vi "RealTime.vi"() -> ()   [LabVIEW 2019]
uses:
  <vilib>/Bytelabs/ByteTCP/TCP_Class/TCP.lvclass
  TypeDef/TCPMessage.ctl
  <vilib>/Bytelabs/ByteSimpleQ/ByteSimpleQ/ByteSimpleQ.lvlib
  TypeDef/ChannelInfo.ctl
  bytetcp/TCPLib/TCP_Class/TCP.lvclass
  <vilib>/Bytelabs/ByteChannelsSetting/ChannelSettingsLib/ChannelsRepos/ChannelsRepoXML/ChannelsRepoXML.lvclass
  source/ByteQXAPIBase/LimsTestStep/acquisitions.ctl
  source/ByteQXAPIBase/ByteQXAPIBase.lvclass
  <vilib>/Utility/xml.llb/Write to XML File(string).vi
  source/ByteQXAPIBase/TypeDef/Step.ctl
  source/ByteQXAPIBase/UpdateChannelsList/fields.ctl
  source/ByteQXAPIBase/TypeDef/Asset.ctl
panel:
  out "error out":errorcluster
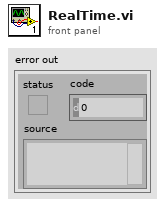
[diagram p1: front panel]
types:
  T1 = typedef "ChannelInfo.ctl" = cluster{"Tag":string, "HW Resource":string, "Raw":dbl}
  T2 = typedef "ByteQXWebAPI.lvlib/ByteQXAPIBase.lvclass/acquisitions.ctl" = cluster{"tags":cluster{"step_id":i32, "test_slug":string, "asset_slug":string}, "acquisitions":cluster{"timestamp":string, "fields":cluster{"name":string, "value":dbl}[]}[]}
  T3 = cluster{"queue out":refnum<queue>, "Acquisitions":T2, "Info":T1[], "TCP_Class":refnum<class "TCP.lvclass">, "Continous?":bool, "Duration":dbl}
  T4 = cluster{"ByteGSAPIBase in":refnum<class "ByteQXAPIBase.lvclass">, "TCP_Class":refnum<class "TCP.lvclass">, "ChannelsRepoBase out":refnum<class "ChannelsRepoXML.lvclass">, "queue out":refnum<queue>}
  T5 = cluster{"ChannelsRepoBase out":refnum<class "ChannelsRepoXML.lvclass">, "channels":string[], "Duration":dbl, "id":i32, "prova.slug":string, "Continous?":bool}
  T6 = cluster{"timestamp":string, "fields":cluster{"name":string, "value":dbl}[]}
  T7 = typedef "TCPMessage.ctl" = cluster{"Message":string, "Data":variant}
  T8 = cluster{"timestamp":string, "fields":cluster{"name":string, "value":dbl}[]}[]
  T9 = typedef "ByteQXWebAPI.lvlib/ByteQXAPIBase.lvclass/fields.ctl" = cluster{"asset_slug":string, "fields":string[]}
  T10 = typedef "ByteQXWebAPI.lvlib/ByteQXAPIBase.lvclass/Step.ctl" = cluster{"id":i32, "descrizione":string, "prova":cluster{"slug":string}, "assets":T11[], "criterio_accettazione":string, "valore_criterio_accettazione_max":dbl, "valore_criterio_accettazione_min":dbl, "udm_criterio_accettazione":string, "duration_prova":string, "udm_duration_prova":string, "valore_prova":dbl, "ordine":i32, "user":i32, "link_automation":string, "instruction_automation":string, "data_completamento_checklist":timestamp, "outcome":bool, "step_type":string, "channels":string[]}
  T11 = typedef "ByteQXWebAPI.lvlib/ByteQXAPIBase.lvclass/Asset.ctl" = cluster{"descrizione":string, "slug":string, "id":i32}
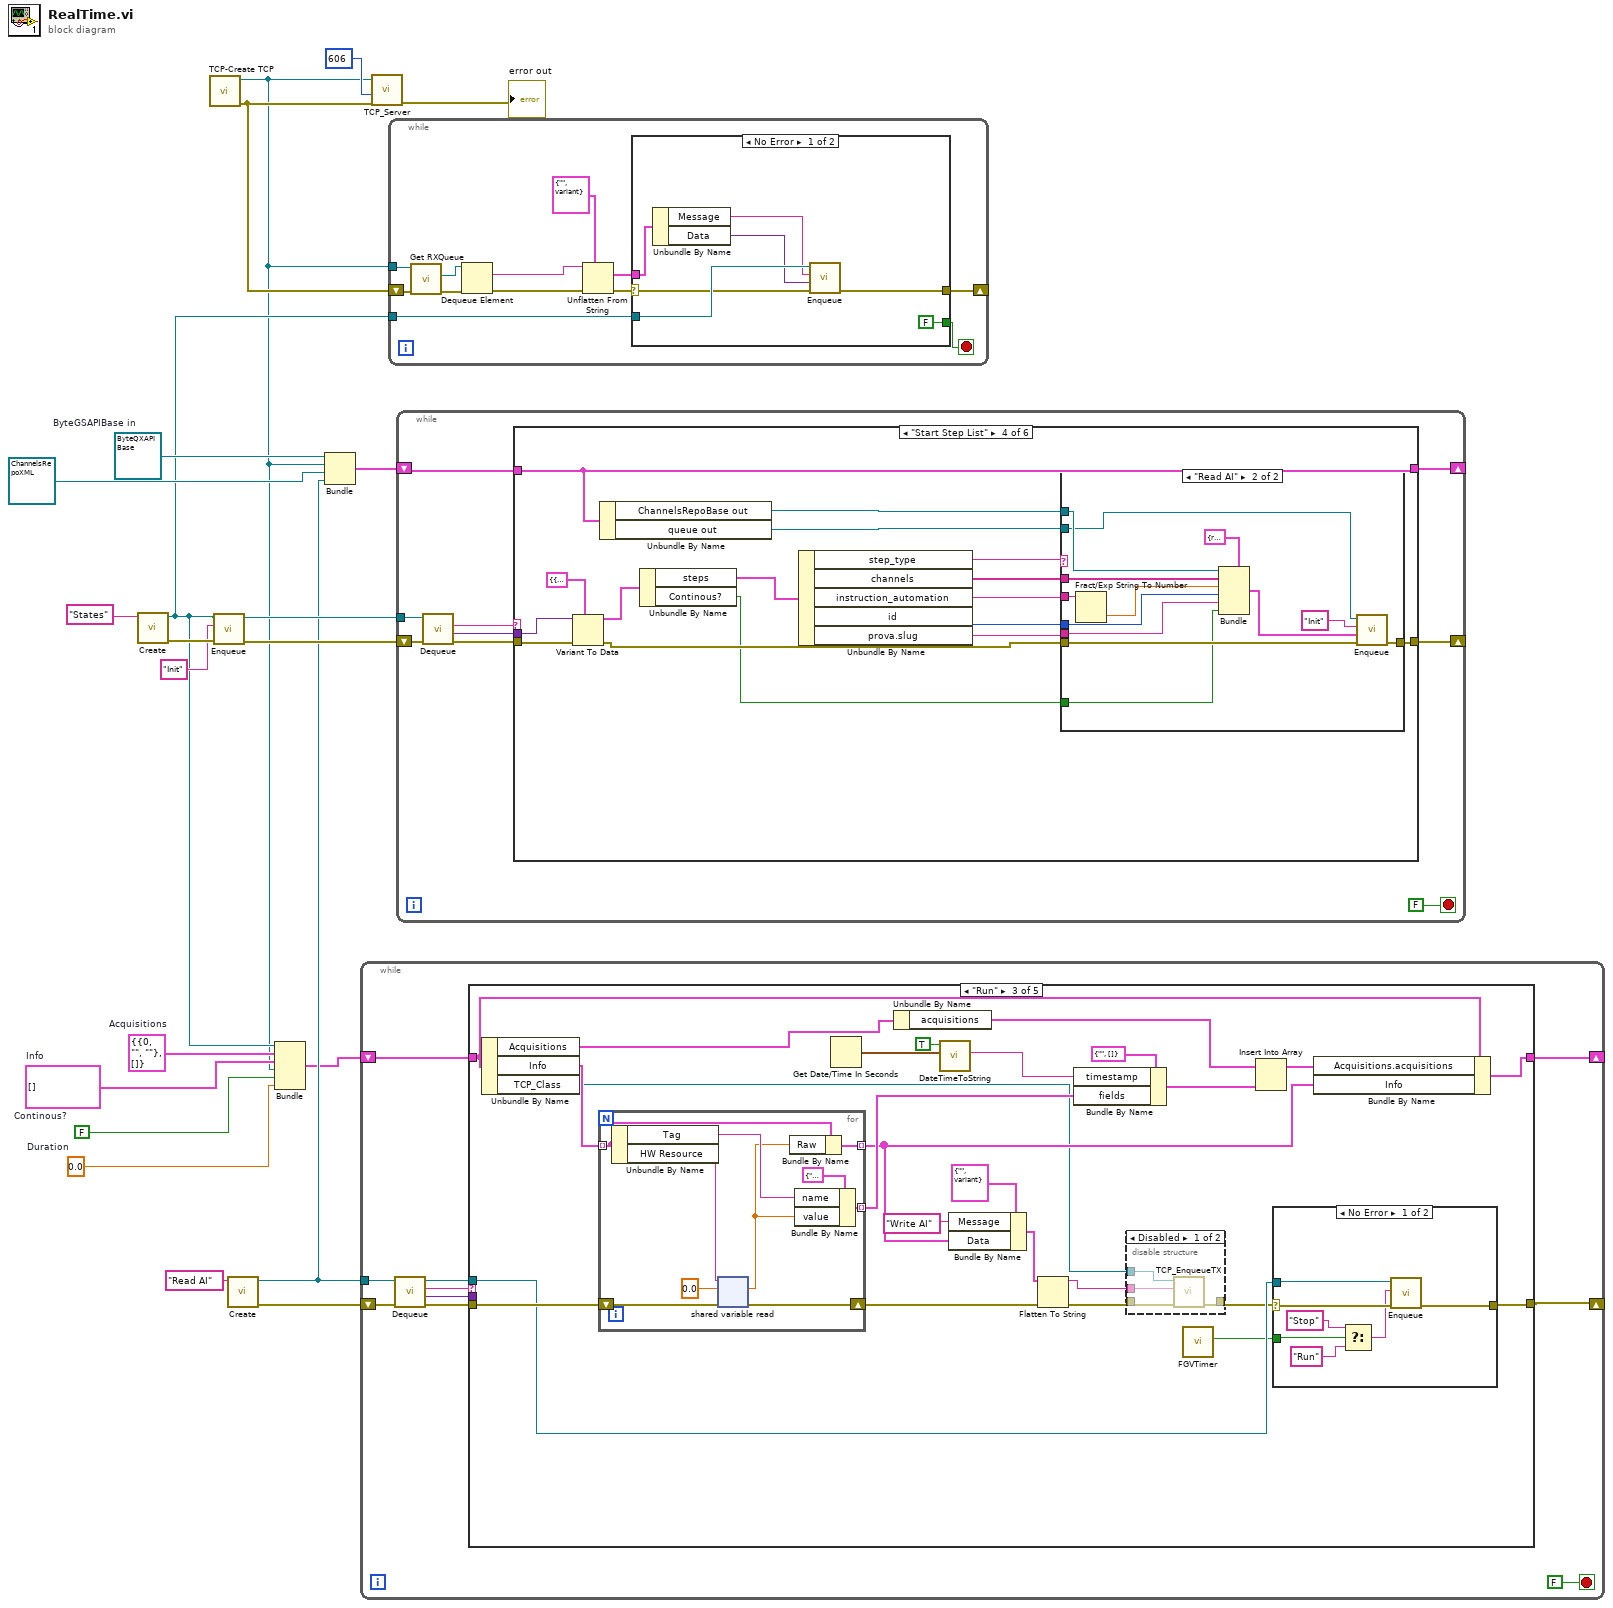
[diagram p0: block diagram]
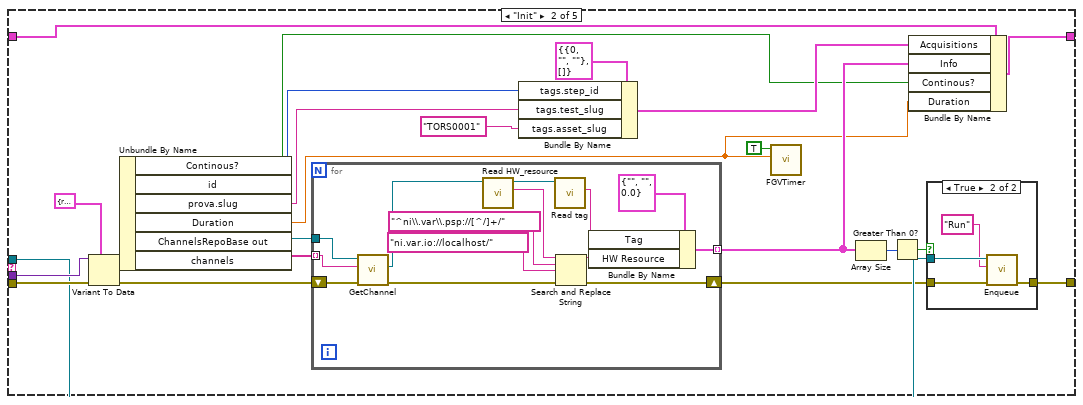
[diagram p3: hidden frame]
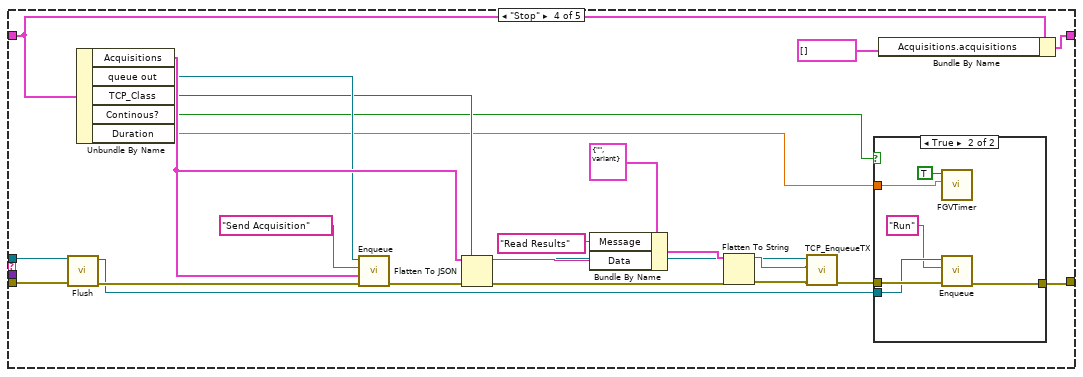
[diagram p7: hidden frame]
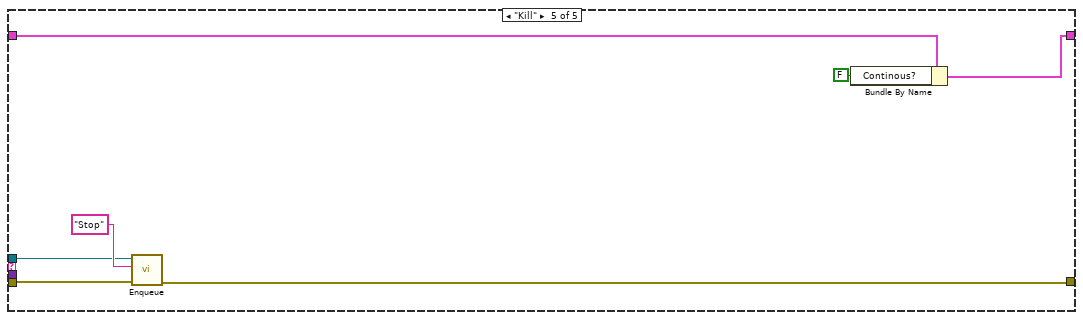
[diagram p9: hidden frame]
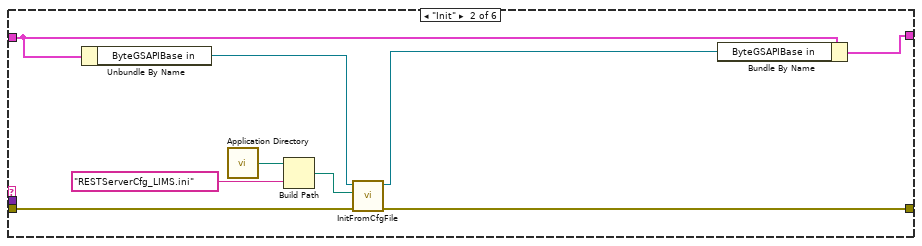
[diagram p11: hidden frame]
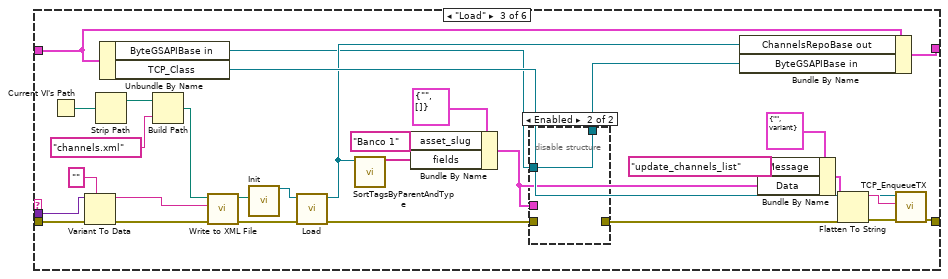
[diagram p12: hidden frame]
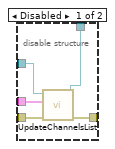
[diagram p13: hidden frame]
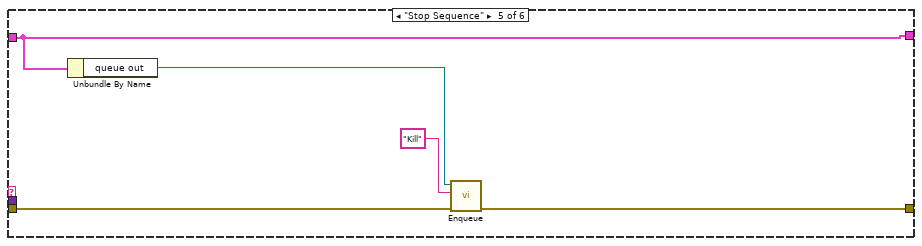
[diagram p15: hidden frame]
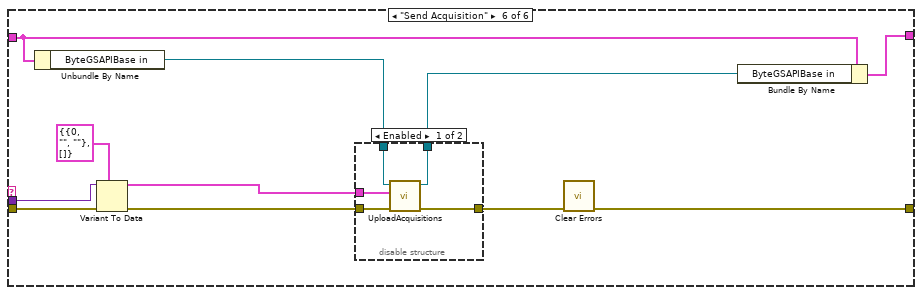
[diagram p16: hidden frame]
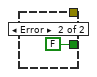
[diagram p18: hidden frame]
diagram:
  w1 = 0.0  # Duration
  w2 = FALSE  # Continous?
  w5 = T1[] []  # Info
  w6 = T2 {"tags"={"step_id"=0, "test_slug"="", "asset_slug"=""}, "acquisitions"=[]}  # Acquisitions
  w11 = refnum<class "ByteQXAPIBase.lvclass"> refnum  # ByteGSAPIBase in
  n1 = call <vilib>:"Create.vi"("name (unnamed)"="States") -> ("error out"=w15:errorcluster, "queue out"=w7:refnum<queue>)  [unwired: 8 in, 1 out]
  n2 = call <vilib>:"TCP-Create TCP.vi"() -> ("error out"=w21:errorcluster, "TCP_Class"=w4:refnum<class "TCP.lvclass">)  [unwired: 9 in, 1 out]
  n3 = call <vilib>:"Enqueue.vi"("error in (no error)"=w15, "message"="Init", "queue in"=w7) -> ("error out"=w14:errorcluster, "queue out"=w13:refnum<queue>)  [unwired: 6 in, 1 out]
  n4 = call <vilib>:"Create.vi"("name (unnamed)"="Read AI") -> ("error out"=w17:errorcluster, "queue out"=w9:refnum<queue>)  [unwired: 8 in, 1 out]
  n5 = Bundle("queue out"=w7, "Acquisitions"=w6, "Info"=w5, "TCP_Class"=w4, "Continous?"=w2, "Duration"=w1) -> (w3:T3)  [unwired: 1 in]
  n6 = Bundle("ByteGSAPIBase in"=w11, "TCP_Class"=w4, "ChannelsRepoBase out"=refnum<class "ChannelsRepoXML.lvclass"> refnum, "queue out"=w9) -> (w8:T4)  [unwired: 1 in]
  n7 = while {
    tunnel: w9 -> [w31]
    shift-right: [w25] -> _
    shift-left: w17 -> [w30]
    shift-right: [w22] -> _
    shift-left: w3 -> [w23]
    stop <- FALSE stop-if-true
    n8 = call <vilib>:"Dequeue.vi"("error in (no error)"=w30, "queue in"=w31) -> ("error out"=w29:errorcluster, "data"=w27:variant, "message"=w28:string, "queue out"=w26:refnum<queue>)  [unwired: 5 in, 1 out]
    n9 = case shown="\"Run\"" w28 {
      tunnel: w29 -> [w33 w56 w100 w145 w158]
      tunnel: w27 -> [_ w55 _ _ _]
      tunnel: w26 -> [_ w51 w99 w144 w157]
      tunnel: [w33 w50 w98 w128 w156] -> w25
      tunnel: w23 -> [w32 w41 w79 w125 w155]
      tunnel: [w32 w39 w77 w124 w153] -> w22
      frame Default {
      }
      frame "Init" {
        n10 = Variant To Data(error in=w56, type=T5 {"ChannelsRepoBase out"=refnum, "channels"=[], "Duration"=0.0, "id"=0, "prova.slug"="", "Continous?"=FALSE} ("output cluster"), Variant=w55) -> (data=w49:T5, error out=w54:errorcluster)
        n11 = Unbundle By Name(w49) -> ("Continous?"=w36:bool, "id"=w43:i32, "prova.slug"=w42:string, "Duration"=w34:dbl, "ChannelsRepoBase out"=w47:refnum<class "ChannelsRepoXML.lvclass">, "channels"=w48:string[])
        n12 = for {
          shift-right: [w70] -> w46
          shift-left: w54 -> [w65]
          tunnel: [w67] -> w38 mode=indexing
          tunnel: w48 -> [w63] mode=indexing
          tunnel: w47 -> [w66]
          n13 = call <vilib>:"GetChannel.vi"("error in (no error)"=w65, "tag"=w63, "ChannelsRepoBase in"=w66) -> ("error out"=w64:errorcluster, "channel"=w62:refnum<class "ChannelBase.lvclass">)  [unwired: 5 in, 2 out]
          n14 = call <vilib>:"Read HW_resource.vi"("ChannelBase in"=w62) -> ("HW_resource"=w75:string, "ChannelBase out"=w72:refnum<class "ChannelBase.lvclass">)  [unwired: 9 in]
          n15 = call <vilib>:"Read tag.vi"("ChannelBase in"=w72) -> ("tag"=w71:string)  [unwired: 9 in, 1 out]
          n16 = Search and Replace String(input string=w75, search string="^ni\\.var\\.psp://[^/]+/", replace string="ni.var.io://localhost/" ("replace string (\"\")"), error in=w64) -> (result string=w69:string, error out=w70:errorcluster)  [unwired: 4 in, 2 out]
          n17 = Bundle By Name(cluster=T1 {"Tag"="", "HW Resource"="", "Raw"=0.0} ("output cluster"), "Tag"=w71, "HW Resource"=w69) -> (w67:T1)
        }
        n18 = Bundle By Name(cluster=T2 {"tags"={"step_id"=0, "test_slug"="", "asset_slug"=""}, "acquisitions"=[]} ("Cluster"), "tags.step_id"=w43, "tags.test_slug"=w42, "tags.asset_slug"="TORS0001") -> (w40:T2)
        n19 = call "FGVTimer.vi"("set timer"=w34, "Reset"=TRUE) -> ()  [unwired: 8 in, 2 out]
        n20 = Array Size(array=w38) -> (size(s)=w53:i32)
        n21 = Greater Than 0?(x=w53) -> (x > 0?=w52:bool)
        n22 = Bundle By Name(cluster=w41, "Acquisitions"=w40, "Info"=w38, "Continous?"=w36, "Duration"=w34) -> (w39:T3)
        n23 = case shown="True" w52 {
          tunnel: w51 -> [_ w61]
          tunnel: [w57 w59] -> w50
          tunnel: w46 -> [w57 w58]
          frame False {
          }
          frame True {
            n24 = call <vilib>:"Enqueue.vi"("error in (no error)"=w58, "message"="Run", "queue in"=w61) -> ("error out"=w59:errorcluster)  [unwired: 6 in, 2 out]
          }
        }
      }
      frame "Run" {
        n25 = Unbundle By Name(w79) -> ("Acquisitions"=w80:T2, "Info"=w81:T1[], "TCP_Class"=w76:refnum<class "TCP.lvclass">)
        n26 = for {
          shift-right: [w118] -> w87
          shift-left: w100 -> [w122]
          tunnel: w81 -> [w119] mode=indexing
          tunnel: [w117] -> w78 mode=indexing
          tunnel: [w114] -> w93 mode=indexing
          n27 = Unbundle By Name(w119) -> ("Tag"=w115:string, "HW Resource"=w120:string)
          n28 = shared-variable-read(w120, w122, 0.0) -> (w118:errorcluster, w113:dbl)  [unwired: 2 out]
          n29 = Bundle By Name(cluster=w119, "Raw"=w113) -> (w117:T1)
          n30 = Bundle By Name(cluster=cluster{"name":string, "value":dbl} {"name"="", "value"=0.0} ("fields"), "name"=w115, "value"=w113) -> (w114:cluster{"name":string, "value":dbl})
        }
        n31 = Get Date/Time In Seconds() -> (seconds since 1Jan1904=w84:timestamp)
        n32 = Unbundle By Name(w80) -> ("acquisitions"=w91:T8)
        n33 = call "DateTimeToString.vi"("current time"=w84, "include Time?"=TRUE) -> ("date string"=w83:string)  [unwired: 8 in, 1 out]
        n34 = Bundle By Name(cluster=T7 {"Message"="", "Data"=variant}, "Message"="Write AI", "Data"=w78) -> (w96:T7)
        n35 = Flatten To String(anything=w96, error in (no error)=w87) -> (data string=w88:string, error out=w89:errorcluster)  [unwired: 2 in, 1 out]
        n36 = Bundle By Name(cluster=T6 {"timestamp"="", "fields"=[]} ("acquisition"), "timestamp"=w83, "fields"=w93) -> (w92:T6)
        n37 = disable-structure shown="Disabled" {
          disable-tunnel: w89 -> [w104 _]
          disable-tunnel: w88 -> [w103 _]
          disable-tunnel: [w102 _] -> w85
          disable-tunnel: w76 -> [w101 _]
          frame Disabled {
            n38 = call-dynamic "TCP_EnqueueTX.vi"("error in (no error)"=w104, "Msg to Transmit"=w103, "TCP in"=w101) -> ("error out"=w102:errorcluster)  [unwired: 7 in, 1 out]
          }
          frame Enabled {
          }
        }
        n39 = call "FGVTimer.vi"() -> ("Elapsed?"=w86:bool)  [unwired: 10 in, 1 out]
        n40 = Insert Into Array(array=w91, new element=w92) -> (w90:T8)  [unwired: 1 in]
        n41 = case shown="No Error" w85 {
          selector: w85 -> [w111 w112]
          tunnel: w99 -> [w109 _]
          tunnel: [w110 w112] -> w98
          tunnel: w86 -> [w108 _]
          frame No Error {
            n42 = Select(t="Stop" ("message"), s=w108, f="Run" ("message")) -> (s? t:f=w105:string)
            n43 = call <vilib>:"Enqueue.vi"("error in (no error)"=w111, "message"=w105, "queue in"=w109) -> ("error out"=w110:errorcluster)  [unwired: 6 in, 2 out]
          }
          frame Error {
          }
        }
        n44 = Bundle By Name(cluster=w79, "Acquisitions.acquisitions"=w90, "Info"=w78) -> (w77:T3)
      }
      frame "Stop" {
        n45 = call <vilib>:"Flush.vi"("error in"=w145, "queue in"=w144) -> ("error out"=w136:errorcluster, "queue out"=w127:refnum<queue>)  [unwired: 8 in]
        n46 = Unbundle By Name(w125) -> ("Acquisitions"=w133:T2, "queue out"=w132:refnum<queue>, "TCP_Class"=w131:refnum<class "TCP.lvclass">, "Continous?"=w130:bool, "Duration"=w126:dbl)
        n47 = call <vilib>:"Enqueue.vi"("error in (no error)"=w136, "data"=w133, "message"="Send Acquisition", "queue in"=w132) -> ("error out"=w135:errorcluster)  [unwired: 5 in, 2 out]
        n48 = Flatten To JSON(anything=w133, error in (no error)=w135) -> (JSON string=w137:string, 11:w138:errorcluster)  [unwired: 1 in]
        n49 = Bundle By Name(cluster=T7 {"Message"="", "Data"=variant}, "Message"="Read Results", "Data"=w137) -> (w142:T7)
        n50 = Flatten To String(anything=w142, error in (no error)=w138) -> (data string=w139:string, error out=w140:errorcluster)  [unwired: 2 in, 1 out]
        n51 = call-dynamic "TCP_EnqueueTX.vi"("error in (no error)"=w140, "Msg to Transmit"=w139, "TCP in"=w131) -> ("error out"=w129:errorcluster)  [unwired: 7 in, 1 out]
        n52 = case shown="True" w130 {
          tunnel: w129 -> [w146 w152]
          tunnel: [w146 w151] -> w128
          tunnel: w127 -> [_ w150]
          tunnel: w126 -> [_ w147]
          frame False {
          }
          frame True {
            n53 = call "FGVTimer.vi"("set timer"=w147, "Reset"=TRUE) -> ()  [unwired: 8 in, 2 out]
            n54 = call <vilib>:"Enqueue.vi"("error in (no error)"=w152, "message"="Run", "queue in"=w150) -> ("error out"=w151:errorcluster)  [unwired: 6 in, 2 out]
          }
        }
        n55 = Bundle By Name(cluster=w125, "Acquisitions.acquisitions"=T8 []) -> (w124:T3)
      }
      frame "Kill" {
        n56 = call <vilib>:"Enqueue.vi"("error in (no error)"=w158, "message"="Stop", "queue in"=w157) -> ("error out"=w156:errorcluster)  [unwired: 6 in, 2 out]
        n57 = Bundle By Name(cluster=w155, "Continous?"=FALSE) -> (w153:T3)
      }
    }
  }
  n58 = call <vilib>:"TCP_Server.vi"("error in (no error)"=w21, "TxPort"=u16 606, "TCP.lvlib:TCP.lvclass"=w4) -> ("error out"=→"error out":errorcluster)  [unwired: 8 in]
  n59 = while {
    tunnel: w4 -> [w163]
    tunnel: w7 -> [w171]
    shift-right: [w167] -> _
    shift-left: w21 -> [w164]
    stop <- w160 stop-if-true
    # "Receiver"
    n60 = call-dynamic "Get RXQueue.vi"("error in (no error)"=w164, "TCP in"=w163) -> ("error out"=w166:errorcluster, "RX"=w165:refnum<queue>)  [unwired: 7 in, 1 out]
    n61 = Dequeue Element(queue=w165, error in (no error)=w166) -> (element=w161:string, error out=w162:errorcluster)  [unwired: 1 in, 2 out]
    n62 = Unflatten From String(type=T7 {"Message"="", "Data"=variant}, binary string=w161, error in (no error)=w162) -> (value=w168:T7, error out=w170:errorcluster)  [unwired: 2 in, 1 out]
    n63 = case shown="No Error" w170 {
      selector: w170 -> [w177 _]
      tunnel: w171 -> [w178 _]
      tunnel: w168 -> [w176 _]
      tunnel: [w173 _] -> w167
      tunnel: [FALSE FALSE] -> w160
      frame No Error {
        n64 = Unbundle By Name(w176) -> ("Message"=w174:string, "Data"=w175:variant)
        n65 = call <vilib>:"Enqueue.vi"("error in (no error)"=w177, "data"=w175, "message"=w174, "queue in"=w178) -> ("error out"=w173:errorcluster)  [unwired: 5 in, 2 out]
      }
      frame Error {
      }
    }
  }
  n66 = while {
    tunnel: w13 -> [w187]
    shift-right: [w182] -> _
    shift-left: w14 -> [w188]
    shift-right: [w180] -> _
    shift-left: w8 -> [w181]
    stop <- FALSE stop-if-true
    n67 = call <vilib>:"Dequeue.vi"("error in (no error)"=w188, "queue in"=w187) -> ("error out"=w186:errorcluster, "data"=w185:variant, "message"=w184:string)  [unwired: 5 in, 2 out]
    n68 = case shown="\"Start Step List\"" w184 {
      tunnel: w186 -> [w190 w199 w221 w251 w269 w281]
      tunnel: w185 -> [_ _ w220 w250 _ w280]
      tunnel: [w190 w198 w215 w247 w268 w275] -> w182
      tunnel: w181 -> [w189 w193 w208 w243 w266 w273]
      tunnel: [w189 w191 w207 w243 w266 w272] -> w180
      frame Default {
      }
      frame "Init" {
        n69 = Unbundle By Name(w193) -> ("ByteGSAPIBase in"=w194:refnum<class "ByteQXAPIBase.lvclass">)
        n70 = call <vilib>:"Application Directory.vi"() -> ("Application Directory"=w196:path)
        n71 = Build Path(base path=w196, name or relative path="RESTServerCfg_LIMS.ini") -> (appended path=w195:path)
        n72 = call-dynamic "InitFromCfgFile.vi"("error in (no error)"=w199, "configuration file path"=w195, "ByteGSAPIBase in"=w194) -> ("error out"=w198:errorcluster, "ByteGSAPIBase out"=w192:refnum<class "ByteQXAPIBase.lvclass">)  [unwired: 7 in]
        n73 = Bundle By Name(cluster=w193, "ByteGSAPIBase in"=w192) -> (w191:T4)
      }
      frame "Load" {
        n74 = Current VI's Path() -> (path=w225:path)
        n75 = Variant To Data(error in=w221, type="", Variant=w220) -> (data=w228:string, error out=w227:errorcluster)
        n76 = Strip Path(path=w225) -> (stripped path=w224:path)  [unwired: 1 out]
        n77 = Unbundle By Name(w208) -> ("ByteGSAPIBase in"=w203:refnum<class "ByteQXAPIBase.lvclass">, "TCP_Class"=w209:refnum<class "TCP.lvclass">)
        n78 = Build Path(base path=w224, name or relative path="channels.xml") -> (appended path=w223:path)
        n79 = call-poly <vilib>:"Write to XML File.vi"("error in (no error)"=w227, "XML Input"=w228, "XML File Path"=w223) -> ("error out"=w219:errorcluster, "XML File Path(duplicate)"=w222:path)  [unwired: 6 in, 1 out]
        n80 = call <vilib>:"Init.vi"("XML file path"=w222) -> ("ChannelsRepoXML out"=w218:refnum<class "ChannelsRepoXML.lvclass">)  [unwired: 10 in]
        n81 = call <vilib>:"Load.vi"("error in (no error)"=w219, "ChannelsRepoBase in"=w218) -> ("error out"=w205:errorcluster, "ChannelsRepoBase out"=w206:refnum<class "ChannelsRepoXML.lvclass">)  [unwired: 7 in, 1 out]
        n82 = call <vilib>:"SortTagsByParentAndType.vi"("ChannelsRepoBase in"=w206) -> ("sorted tags"=w216:string[])  [unwired: 8 in, 2 out]
        n83 = Bundle By Name(cluster=T9 {"asset_slug"="", "fields"=[]} ("Channels"), "asset_slug"="Banco 1", "fields"=w216) -> (w202:T9)
        n84 = disable-structure shown="Enabled" {
          disable-tunnel: w205 -> [w234 _]
          disable-tunnel: [w233 _] -> w204
          disable-tunnel: w203 -> [w232 w235]
          disable-tunnel: w202 -> [w231 _]
          disable-tunnel: [w230 w235] -> w201
          frame Disabled {
            n85 = call "UpdateChannelsList.vi"("error in (no error)"=w234, "Channels"=w231, "ByteGSAPIBase in"=w232) -> ("error out"=w233:errorcluster, "ByteGSAPIBase out"=w230:refnum<class "ByteGSAPIBase.lvclass">)  [unwired: 7 in]
          }
          frame Enabled {
          }
        }
        n86 = Bundle By Name(cluster=w208, "ChannelsRepoBase out"=w206, "ByteGSAPIBase in"=w201) -> (w207:T4)
        n87 = Bundle By Name(cluster=T7 {"Message"="", "Data"=variant} ("Cluster"), "Message"="update_channels_list", "Data"=w202) -> (w211:T7)
        n88 = Flatten To String(anything=w211, error in (no error)=w204) -> (data string=w210:string, error out=w212:errorcluster)  [unwired: 2 in, 1 out]
        n89 = call-dynamic "TCP_EnqueueTX.vi"("error in (no error)"=w212, "Msg to Transmit"=w210, "TCP in"=w209) -> ("error out"=w215:errorcluster)  [unwired: 7 in, 1 out]
      }
      frame "Start Step List" {
        n90 = Variant To Data(error in=w251, type=cluster{"steps":T10, "Continous?":bool} {"steps"={"id"=0, "descrizione"="", "prova"={"slug"=""}, "assets"=[], "criterio_accettazione"="", "valore_criterio_accettazione_max"=0.0, "valore_criterio_accettazione_min"=0.0, "udm_criterio_accettazione"="", "duration_prova"="", "udm_duration_prova"="", "valore_prova"=0.0, "ordine"=0, "user"=0, "link_automation"="", "instruction_automation"="", "data_completamento_checklist"=timestamp(0 s since 1904-01-01), "outcome"=FALSE, "step_type"="", "channels"=[]}, "Continous?"=FALSE}, Variant=w250) -> (data=w238:cluster{"steps":T10, "Continous?":bool}, error out=w248:errorcluster)
        n91 = Unbundle By Name(w243) -> ("ChannelsRepoBase out"=w244:refnum<class "ChannelsRepoXML.lvclass">, "queue out"=w242:refnum<queue>)
        n92 = Unbundle By Name(w238) -> ("steps"=w237:T10, "Continous?"=w236:bool)
        n93 = Unbundle By Name(w237) -> ("step_type"=w249:string, "channels"=w246:string[], "instruction_automation"=w245:string, "id"=w241:i32, "prova.slug"=w240:string)
        n94 = case shown="\"Read AI\"" w249 {
          tunnel: w248 -> [w252 w265]
          tunnel: [w252 w264] -> w247
          tunnel: w246 -> [_ w262]
          tunnel: w245 -> [_ w260]
          tunnel: w244 -> [_ w257]
          tunnel: w242 -> [_ w256]
          tunnel: w241 -> [_ w255]
          tunnel: w240 -> [_ w254]
          tunnel: w236 -> [_ w253]
          frame Default {
          }
          frame "Read AI" {
            n95 = Fract/Exp String To Number(string=w260) -> (number=w259:dbl)  [unwired: 3 in, 1 out]
            n96 = Bundle(cluster=T5 {"ChannelsRepoBase out"=refnum, "channels"=[], "Duration"=0.0, "id"=0, "prova.slug"="", "Continous?"=FALSE} ("output cluster"), "ChannelsRepoBase out"=w257, "channels"=w262, "Duration"=w259, "id"=w255, "prova.slug"=w254, "Continous?"=w253) -> (w261:T5)
            n97 = call <vilib>:"Enqueue.vi"("error in (no error)"=w265, "data"=w261, "message"="Init", "queue in"=w256) -> ("error out"=w264:errorcluster)  [unwired: 5 in, 2 out]
          }
        }
      }
      frame "Stop Sequence" {
        n98 = Unbundle By Name(w266) -> ("queue out"=w267:refnum<queue>)
        n99 = call <vilib>:"Enqueue.vi"("data"=w269, "message"="Kill", "queue in"=w267) -> ("error out"=w268:errorcluster)  [unwired: 6 in, 2 out]
      }
      frame "Send Acquisition" {
        n100 = Unbundle By Name(w273) -> ("ByteGSAPIBase in"=w274:refnum<class "ByteQXAPIBase.lvclass">)
        n101 = Variant To Data(error in=w281, type=T2 {"tags"={"step_id"=0, "test_slug"="", "asset_slug"=""}, "acquisitions"=[]} ("Acquisitions"), Variant=w280) -> (data=w277:T2, error out=w278:errorcluster)
        n102 = disable-structure shown="Enabled" {
          disable-tunnel: w274 -> [w286 _]
          disable-tunnel: w278 -> [w285 _]
          disable-tunnel: w277 -> [w284 _]
          disable-tunnel: [w283 _] -> w271
          disable-tunnel: [w282 _] -> w276
          frame Enabled {
            n103 = call-dynamic "UploadAcquisitions.vi"("error in (no error)"=w285, "Acquisitions"=w284, "ByteGSAPIBase in"=w286) -> ("error out"=w282:errorcluster, "ByteGSAPIBase out"=w283:refnum<class "ByteQXAPIBase.lvclass">)  [unwired: 7 in]
          }
          frame Disabled {
          }
        }
        n104 = call <vilib>:"Clear Errors.vi"("error in (no error)"=w276) -> ("error out"=w275:errorcluster)  [unwired: 5 in, 1 out]
        n105 = Bundle By Name(cluster=w273, "ByteGSAPIBase in"=w271) -> (w272:T4)
      }
    }
  }
